vi "Fast_PID_with_Slow_Logging.vi"() -> ()   [LabVIEW 2018]
uses:
  SendStuff/SlowLogger.lvclass
  SendStuff/SlowLogger.lvclass/SlowLogger.ctl
  84b83d19-6426-4179-911e-7fff3597e1d2.vi
  84b83d19-6426-4179-911e-7fff3597e1d2.vi/dd311a3f-021d-468f-a0ef-81a33d201e34.vi
  SendStuff/SlowLogger_LogThisSlowly.vi/f93abad2-5217-430f-97d3-b2f2641e9ea3.vi
  SendStuff/SlowLogger_LogThisSlowly.vi/f93abad2-5217-430f-97d3-b2f2641e9ea3.vi/d3fdaf2b-79b9-493c-b5bc-ddf1d10edc78.vi
  feGEM DataPacker.lvlib
panel:
  in  "MIDAS Sever Port":u16=12345
  in  "MIDAS Server":string="my_midas_server.domain"
  out "error out":errorcluster
  out "Dt (s) 2":dbl
  out "Dt (s)":dbl
  out "Variable Rate Array\nDt satisfied (data logged) 2":bool=TRUE
  out "Slow Logging Array\nDt satisfied (data logged)":bool=TRUE
  out "error out":errorcluster
  in  "Slow Logging Array":dbl[](array[numeric])=[0.1, 0.2, 0.3, 0.4, 0.5, 0.6, 0.7, 0.8, 0.9, 1.0]
  in  "Variable Rate Array (Logs faster if sum >10)":dbl[](array[numeric])=[0.1, 0.2, 0.3, 0.4, 0.5, 0.6, 0.7, 0.8, 0.9, 1.0]
  out "Announcement Error":errorcluster
  in  "stop":bool
  out "error out":errorcluster
  in  "Temperature array":dbl[](array[numeric])=[0.1, 0.2, 0.3, 0.4, 0.5, 0.6, 0.7, 0.8, 0.9, 1.0]
  out "Get Run Status Error out":errorcluster
  out "Run Status":string
  out "Get RunNumber Error out":errorcluster
  out "RUNNO":i32
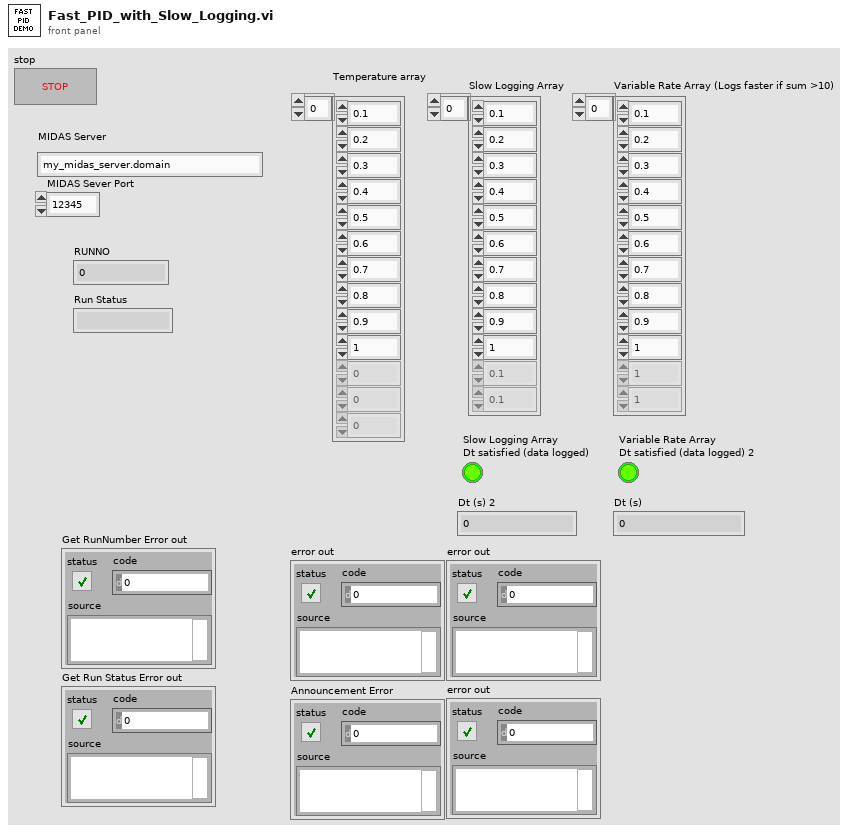
[diagram p1: front panel]
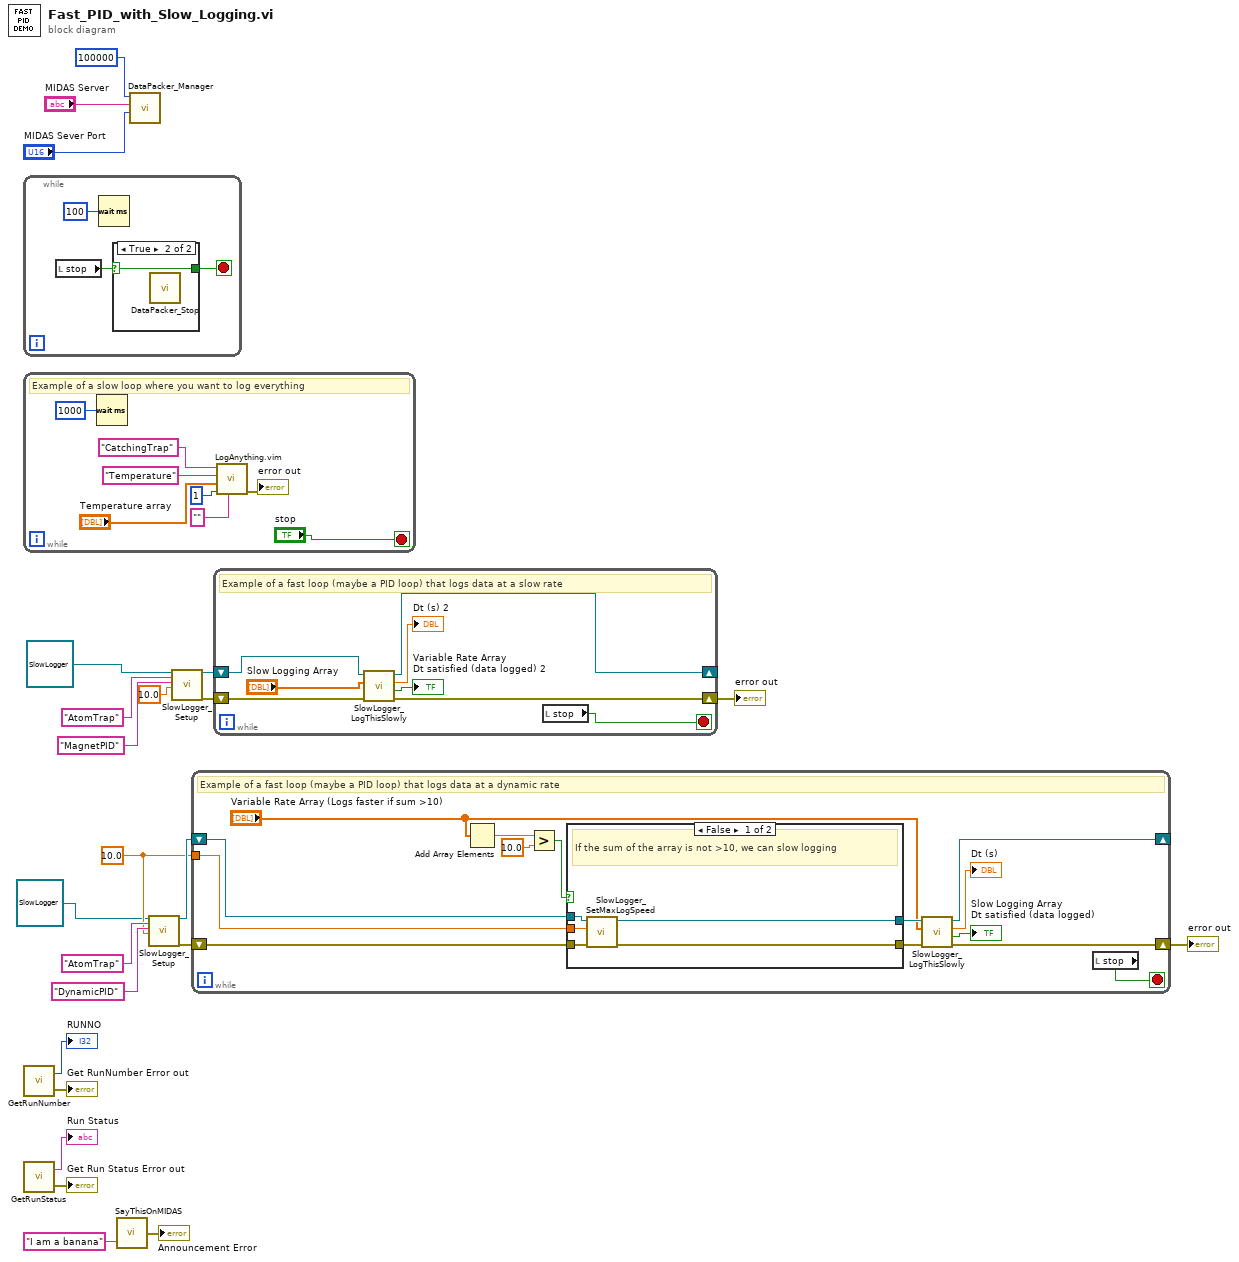
[diagram p0: block diagram]
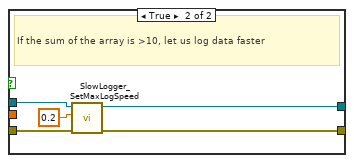
[diagram p3: hidden frame]
diagram:
  w7 = 10.0 ("Max Log Speed (HZ)")
  n1 = while {
    stop <- w25 stop-if-true
    n2 = local read "stop"() -> (w24:bool)
    n3 = Wait (ms)(milliseconds to wait=u32 100) -> ()  [unwired: 1 out]
    n4 = case shown="True" w24 {
      selector: w24 -> [w27 w28]
      tunnel: [w27 w28] -> w25
      frame False {
      }
      frame True {
        n5 = call "DataPacker_Stop.vi"() -> ()  [unwired: 12 in]
      }
    }
  }
  n6 = while {
    stop <- "stop" stop-if-true
    # "Example of a slow loop where you want to log everything"
    n7 = Wait (ms)(milliseconds to wait=u32 1000) -> ()  [unwired: 1 out]
    n8 = call "LogAnything.vim"("Equipment description (32 chars)"="" ("Equipment description"), "Period to update history plots (seconds)\nUnset (65535) = Use MIDAS default in ODB\n0 = Record but do not put in histories"=1 ("Rate to update history plots"), "Array"="Temperature array", "Variable Name"="Temperature" ("Var Name"), "Category"="CatchingTrap") -> ("error out"=→"error out":errorcluster)  [unwired: 6 in]
  }
  n9 = call "GetRunNumber.vi"() -> ("error out"=→"Get RunNumber Error out":errorcluster, "RunNumber"=→"RUNNO":i32)  [unwired: 2 in]
  n10 = call "GetRunStatus.vi"() -> ("error out"=→"Get Run Status Error out":errorcluster, "Run Status"=→"Run Status":string)  [unwired: 2 in]
  n11 = call "SayThisOnMIDAS.vi"("String"="I am a banana") -> ("error out"=→"Announcement Error":errorcluster)  [unwired: 1 in]
  n12 = call "DataPacker_Manager.vi"("MIDAS Sever Port"="MIDAS Sever Port", "MIDAS Server"="MIDAS Server", "Override Max Event size (Data rate bytes/s). Use MIDAS Default = 0"=u32 100000 ("Override Max Event size (Data rate kb/s). Use MIDAS Default = 0")) -> ()  [unwired: 9 in]
  n13 = call "SlowLogger_Setup.vi"("SlowLogger in"=refnum<class "SlowLogger.lvclass"> refnum ("feGEM DataPacker.lvlib:SlowLogger.lvclass"), "Category"="AtomTrap", "Variable Name"="DynamicPID", "Max Log Speed [Delta Time] (seconds)"=w7) -> ("SlowLogger out"=w10:refnum<class "SlowLogger.lvclass">, "error out"=w9:errorcluster)  [unwired: 14 in]
  n14 = call "SlowLogger_Setup.vi"("SlowLogger in"=refnum<class "SlowLogger.lvclass"> refnum ("feGEM DataPacker.lvlib:SlowLogger.lvclass"), "Category"="AtomTrap", "Variable Name"="MagnetPID", "Max Log Speed [Delta Time] (seconds)"=10.0 ("Max Log Speed (HZ)")) -> ("SlowLogger out"=w14:refnum<class "SlowLogger.lvclass">, "error out"=w13:errorcluster)  [unwired: 14 in]
  n15 = while {
    shift-right: [w44] -> _
    shift-left: w10 -> [w49]
    shift-right: [w42] -> w8
    shift-left: w9 -> [w48]
    tunnel: w7 -> [w41]
    stop <- w37 stop-if-true
    # "Example of a fast loop (maybe a PID loop) that logs data at a dynamic rate"
    n16 = Add Array Elements(numeric array="Variable Rate Array (Logs faster if sum >10)") -> (sum=w45:dbl)
    n17 = Greater?(x=w45, y=10.0) -> (0:w46:bool)
    n18 = case shown="False" w46 {
      tunnel: [w55 w59] -> w50
      tunnel: w49 -> [w54 w60]
      tunnel: w48 -> [w52 w57]
      tunnel: [w53 w56] -> w43
      tunnel: w41 -> [w51 _]
      frame False {
        # "If the sum of the array is not >10, we can slow logging"
        n19 = call "SlowLogger_SetMaxLogSpeed.vi"("error in (no error)"=w52, "Max Log Speed [Delta Time] (seconds)"=w51, "SlowLogger in"=w54) -> ("error out"=w53:errorcluster, "SlowLogger out"=w55:refnum<class "SlowLogger.lvclass">)  [unwired: 7 in]
      }
      frame True {
        # "If the sum of the array is >10, let us log data faster"
        n20 = call "SlowLogger_SetMaxLogSpeed.vi"("error in (no error)"=w57, "Max Log Speed [Delta Time] (seconds)"=0.2, "SlowLogger in"=w60) -> ("error out"=w56:errorcluster, "SlowLogger out"=w59:refnum<class "SlowLogger.lvclass">)  [unwired: 7 in]
      }
    }
    n21 = call "SlowLogger_LogThisSlowly.vi"("error in (no error)"=w43, "Array"="Variable Rate Array (Logs faster if sum >10)", "SlowLogger in"=w50) -> ("error out"=w42:errorcluster, "Dt satisfied (data logged)"=→"Slow Logging Array\nDt satisfied (data logged)":bool, "Dt (s)"=→"Dt (s)":dbl, "SlowLogger out"=w44:refnum<class "SlowLogger.lvclass">)  [unwired: 5 in]
    n22 = local read "stop"() -> (w37:bool)
  }
  "error out" <- w8
  n23 = while {
    shift-right: [w63] -> _
    shift-left: w14 -> [w68]
    shift-right: [w62] -> w6
    shift-left: w13 -> [w67]
    stop <- w61 stop-if-true
    # "Example of a fast loop (maybe a PID loop) that logs data at a slow rate"
    n24 = call "SlowLogger_LogThisSlowly.vi"("error in (no error)"=w67, "Array"="Slow Logging Array", "SlowLogger in"=w68) -> ("error out"=w62:errorcluster, "Dt satisfied (data logged)"=→"Variable Rate Array\nDt satisfied (data logged) 2":bool, "Dt (s)"=→"Dt (s) 2":dbl, "SlowLogger out"=w63:refnum<class "SlowLogger.lvclass">)  [unwired: 5 in]
    n25 = local read "stop"() -> (w61:bool)
  }
  "error out" <- w6
